vi "Ballard - 1553 - Message.vi"(8 "error in (no error)":errorcluster, 11 "Node Ptr":T2 format="%.0x") -> (0 "error out":errorcluster)   [LabVIEW 2020, in "Ballard 1553 System Explorer.lvlib"]
uses:
  Ballard 1553 System Explorer.lvlib
  <vilib>/NI VeriStand/Custom Device API/Custom Device API.lvlib
  Shared/Controls and Global/Global.vi
  Shared/Ballard 1553 Shared.lvlib
  SubVIs/Parse XML Ballard/Ballard_messageType.ctl
  <vilib>/NI VeriStand/Custom Device API/Get Item Property (Variant).vi
  SubVIs/Parse XML Ballard/Ballard_CWD1.ctl
  SubVIs/Parse XML Ballard/Ballard_CWD2.ctl
  <vilib>/NI VeriStand/Custom Device API/Get Item Property (U16).vi
  <vilib>/NI VeriStand/Custom Device API/Custom Device Item Ref.ctl
panel:
  out "TA2":i8 caption="Terminal Address (TA 2)"
  out "SA2":i8 caption="Terminal Sub-Address (SA 2)"
  out "MC":i8 caption="Mode Code (MC)"
  out "WC":i8 caption="Words Count (WC)"
  out "SA1":i8 caption="Terminal Sub-Address (SA 1)"
  out "TA1":i8 caption="Terminal Address (TA 1)"
  out "Message Type":T1
  in  "Header":cluster{"Section Name":string}={"Section Name"="Ballard - MIL-STD-1553 - Custom Device - Message"}
  in  "Description":string
  out "Name":string
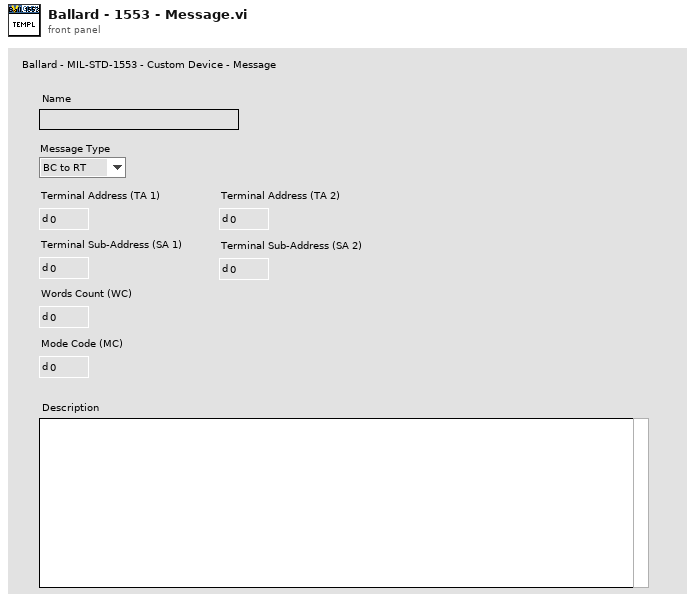
[diagram p1: front panel]
types:
  T1 = typedef "Ballard 1553 System Explorer.lvlib/Ballard_messageType.ctl" = enum16{"BC to RT", "RT to BC", "RT to RT", "MC (Rx)", "MC (Tx)"}
  T2 = typedef "Custom Device API.lvlib/Custom Device Item Ref.ctl" = u64
  T3 = typedef "Ballard 1553 System Explorer.lvlib/Ballard_CWD2.ctl" = cluster{"TA (RT)":i8, "SA":i8, "Words (WC)":i8}
  T4 = typedef "Ballard 1553 System Explorer.lvlib/Ballard_CWD1.ctl" = cluster{"TA (RT)":i8, "SA":i8, "Mode Code":i8, "Words Count":i8}
  T5 = typedef "Custom Device API.lvlib/Custom Device Item Info.ctl" = cluster{"Name":string, "Is Channel":bool, "GUID":string, "Is Waveform":bool}
  T6 = typedef "Custom Device API.lvlib/Custom Device Commands.ctl" = enum16{"Default", "Item renamed", "Shutdown", "Dynamic button pressed"}
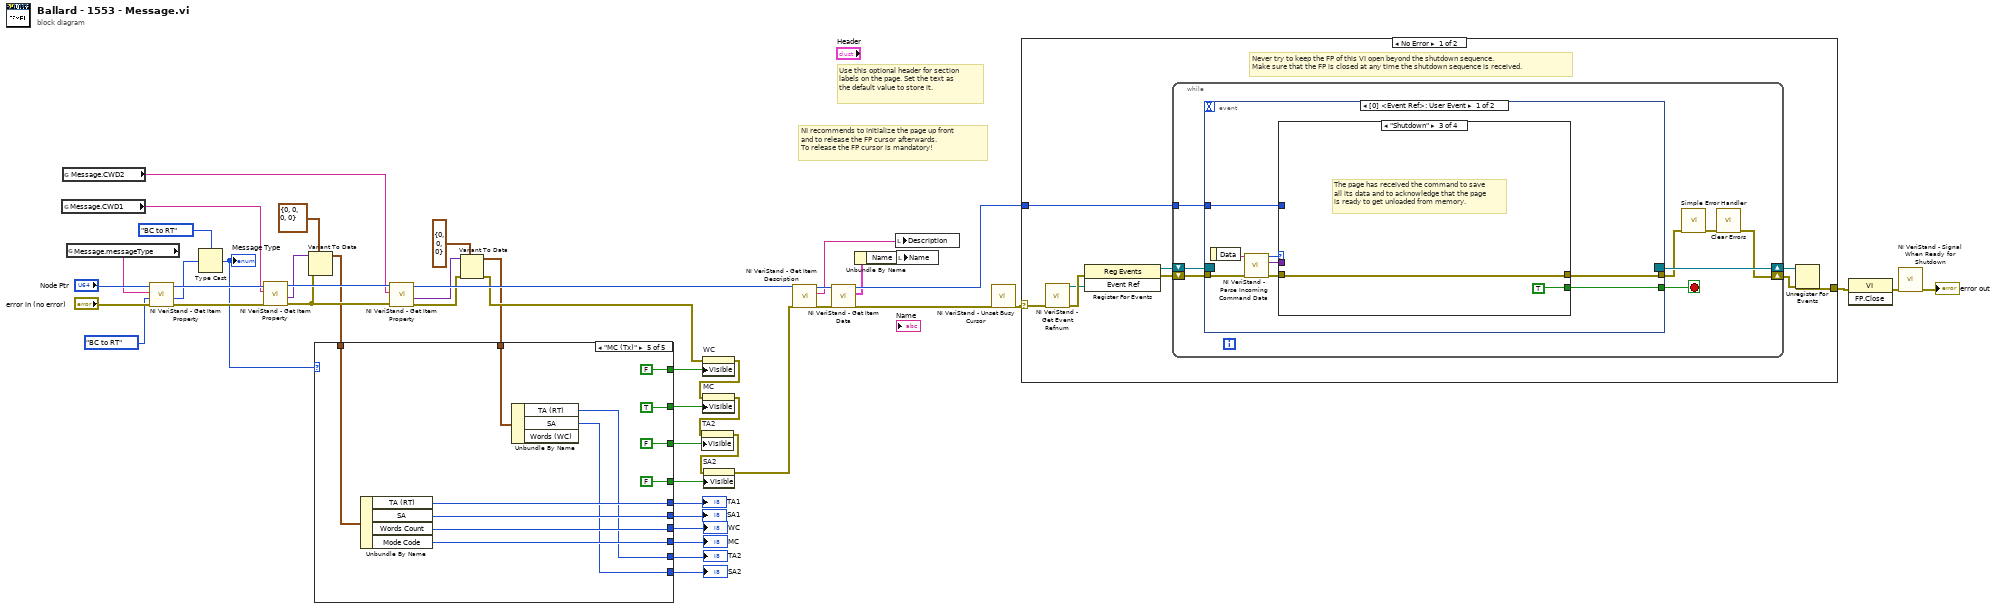
[diagram p0: block diagram]
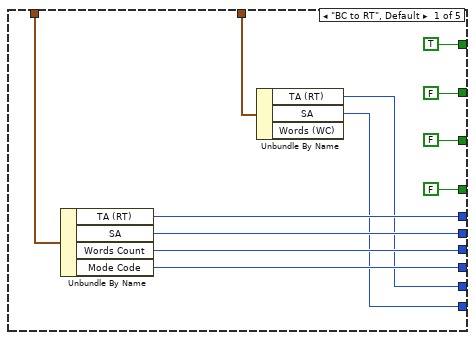
[diagram p2: hidden frame]
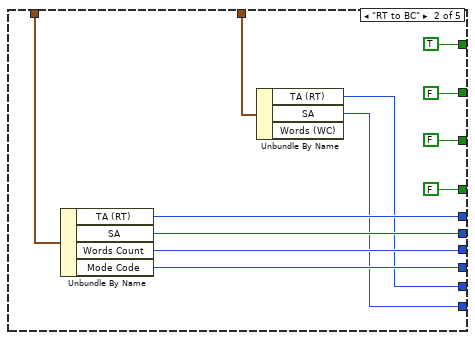
[diagram p3: hidden frame]
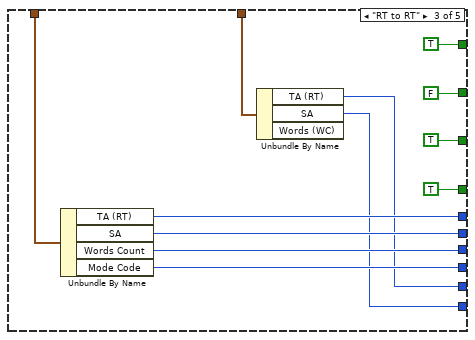
[diagram p4: hidden frame]
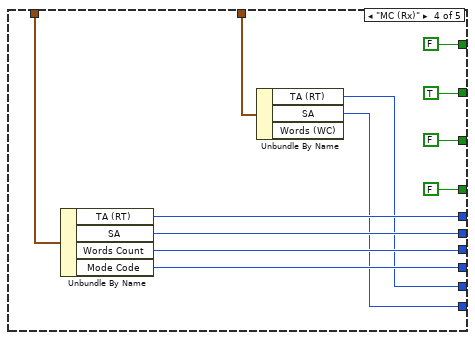
[diagram p5: hidden frame]
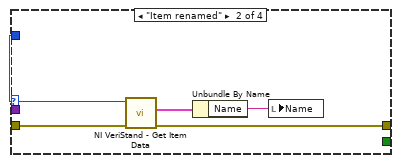
[diagram p7: hidden frame]
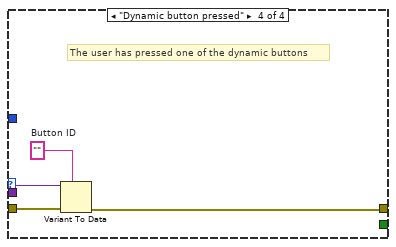
[diagram p8: hidden frame]
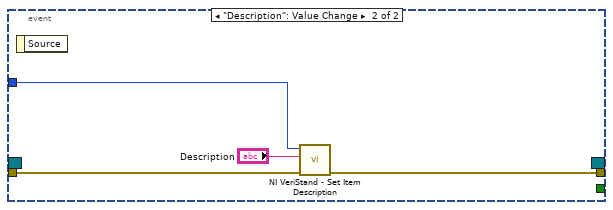
[diagram p9: hidden frame]
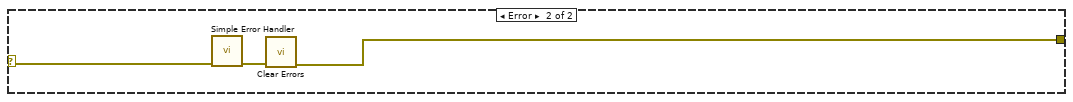
[diagram p10: hidden frame]
diagram:
  # "Use this optional header for section labels on the page. Set the text as the default value to store it."
  # "NI recommends to initialize the page up front\nand to release the FP cursor afterwards.\nTo release the FP cursor is mandatory!"
  n1 = global read "Global.vi" "Message.CWD1"() -> (w27:string)
  n2 = global read "Global.vi" "Message.CWD2"() -> (w21:string)
  n3 = global read "Global.vi" "Message.messageType"() -> (w31:string)
  n4 = call-poly <vilib>:"NI VeriStand - Get Item Property.vi"("error in (no error)"="error in (no error)", "Default Value"=Ballard_messageType."BC to RT" ("messageType"), "Property Name"=w31, "Item Ref in"="Node Ptr") -> ("error out"=w35:errorcluster, "Value"=w30:u16, "Item Ref out"=w32:T2)  [unwired: 4 in, 1 out]
  n5 = Type Cast(type=Ballard_messageType."BC to RT" ("messageType"), x=w30) -> (*(type *) &x=w18:T1)
  "Message Type" <- w18
  n6 = call-poly <vilib>:"NI VeriStand - Get Item Property.vi"("error in (no error)"=w35, "Property Name"=w27, "Item Ref in"=w32) -> ("error out"=w26:errorcluster, "Value"=w25:variant, "Item Ref out"=w36:T2)  [unwired: 5 in, 1 out]
  n7 = Variant To Data(error in=w26, type=T4 {"TA (RT)"=0, "SA"=0, "Mode Code"=0, "Words Count"=0} ("CWD1"), Variant=w25) -> (data=w12:T4)  [unwired: 1 out]
  n8 = call-poly <vilib>:"NI VeriStand - Get Item Property.vi"("error in (no error)"=w26, "Property Name"=w21, "Item Ref in"=w36) -> ("error out"=w20:errorcluster, "Value"=w19:variant, "Item Ref out"=w23:T2)  [unwired: 5 in, 1 out]
  n9 = Variant To Data(error in=w20, type=T3 {"TA (RT)"=0, "SA"=0, "Words (WC)"=0} ("CWD1"), Variant=w19) -> (data=w11:T3, error out=w17:errorcluster)
  n10 = case shown="\"MC (Tx)\"" w18 {
    tunnel: w12 -> [w55 w67 w79 w91 w103]
    tunnel: w11 -> [w50 w62 w74 w86 w98]
    tunnel: [FALSE FALSE TRUE FALSE FALSE] -> w10
    tunnel: [FALSE FALSE TRUE FALSE FALSE] -> w9
    tunnel: [FALSE FALSE FALSE TRUE TRUE] -> w8
    tunnel: [TRUE TRUE TRUE FALSE FALSE] -> w7
    tunnel: [w54 w66 w78 w90 w102] -> w6
    tunnel: [w53 w65 w77 w89 w101] -> w5
    tunnel: [w52 w64 w76 w88 w100] -> w4
    tunnel: [w51 w63 w75 w87 w99] -> w3
    tunnel: [w49 w61 w73 w85 w97] -> w2
    tunnel: [w48 w60 w72 w84 w96] -> w1
    frame "BC to RT", Default {
      n11 = Unbundle By Name(w55) -> ("TA (RT)"=w54:i8, "SA"=w53:i8, "Words Count"=w52:i8, "Mode Code"=w51:i8)
      n12 = Unbundle By Name(w50) -> ("TA (RT)"=w49:i8, "SA"=w48:i8)  [unwired: 1 out]
    }
    frame "RT to BC" {
      n13 = Unbundle By Name(w67) -> ("TA (RT)"=w66:i8, "SA"=w65:i8, "Words Count"=w64:i8, "Mode Code"=w63:i8)
      n14 = Unbundle By Name(w62) -> ("TA (RT)"=w61:i8, "SA"=w60:i8)  [unwired: 1 out]
    }
    frame "RT to RT" {
      n15 = Unbundle By Name(w79) -> ("TA (RT)"=w78:i8, "SA"=w77:i8, "Words Count"=w76:i8, "Mode Code"=w75:i8)
      n16 = Unbundle By Name(w74) -> ("TA (RT)"=w73:i8, "SA"=w72:i8)  [unwired: 1 out]
    }
    frame "MC (Rx)" {
      n17 = Unbundle By Name(w91) -> ("TA (RT)"=w90:i8, "SA"=w89:i8, "Words Count"=w88:i8, "Mode Code"=w87:i8)
      n18 = Unbundle By Name(w86) -> ("TA (RT)"=w85:i8, "SA"=w84:i8)  [unwired: 1 out]
    }
    frame "MC (Tx)" {
      n19 = Unbundle By Name(w103) -> ("TA (RT)"=w102:i8, "SA"=w101:i8, "Words Count"=w100:i8, "Mode Code"=w99:i8)
      n20 = Unbundle By Name(w98) -> ("TA (RT)"=w97:i8, "SA"=w96:i8)  [unwired: 1 out]
    }
  }
  "TA1" <- w6
  "SA1" <- w5
  "WC" <- w4
  "MC" <- w3
  "TA2" <- w2
  "SA2" <- w1
  n21 = property on="WC" class="DigNum (strict)"(error in=w17, "Visible"=w7) -> (error out=w16:errorcluster)  [unwired: 1 in, 1 out]
  n22 = property on="MC" class="DigNum (strict)"(error in=w16, "Visible"=w8) -> (error out=w15:errorcluster)  [unwired: 1 in, 1 out]
  n23 = property on="TA2" class="DigNum (strict)"(error in=w15, "Visible"=w10) -> (error out=w14:errorcluster)  [unwired: 1 in, 1 out]
  n24 = property on="SA2" class="DigNum (strict)"(error in=w14, "Visible"=w9) -> (error out=w13:errorcluster)  [unwired: 1 in, 1 out]
  n25 = call <vilib>:"NI VeriStand - Get Item Description.vi"("error in (no error)"=w13, "Item Ref in"=w23) -> ("error out"=w39:errorcluster, "Description"=w40:string, "Item Ref out"=w41:T2)  [unwired: 7 out]
  n26 = call <vilib>:"NI VeriStand - Get Item Data.vi"("error in (no error)"=w39, "Item Ref in"=w41) -> ("error out"=w44:errorcluster, "Item Info"=w38:T5, "Item Ref out"=w42:T2)  [unwired: 7 out]
  n27 = Unbundle By Name(w38) -> ("Name"=w37:string)
  n28 = local write "Description"(w40) -> ()
  n29 = local write "Name"(w37) -> ()
  n30 = call <vilib>:"NI VeriStand - Unset Busy Cursor.vi"("error in (no error)"=w44) -> ("error out"=w43:errorcluster)  [unwired: 10 out]
  n31 = case shown="No Error" w43 {
    selector: w43 -> [w108 w151]
    tunnel: [w113 w149] -> w47
    tunnel: w42 -> [w109 _]
    frame No Error {
      # "Never try to keep the FP of this VI open beyond the shutdown sequence.\nMake sure that the FP is closed at any time the shutdown sequence is received."
      n32 = call <vilib>:"NI VeriStand - Get Event Refnum.vi"("error in (no error)"=w108) -> ("error out"=w116:errorcluster, "Event Ref"=w112:refnum<user-event>)  [unwired: 9 out]
      n33 = register-events(error in=w116, w112) -> (reference out=w110:refnum<event-registration>, error out=w111:errorcluster)  [unwired: 1 in]
      n34 = while {
        tunnel: w109 -> [w120]
        shift-right: [w117] -> w114
        shift-left: w111 -> [w123]
        shift-right: [w124] -> w115
        shift-left: w110 -> [w122]
        stop <- w121 stop-if-true
        n35 = event shown="[0] <Event Ref>: User Event" {
          selector: w122 -> [_ _]
          dyn-events: [_ _] -> w124
          timeout: _ -> [_ _]
          tunnel: w123 -> [w132 w147]
          tunnel: [w128 _] -> w121
          tunnel: [w127 w146] -> w119
          tunnel: w120 -> [w126 w148]
          event User Event {
            n36 = event-data() -> ("Data"=w131:string)  [unwired: 1 out]
            n37 = call <vilib>:"NI VeriStand - Parse Incoming Command Data.vi"("error in (no error)"=w132, "Incoming data"=w131) -> ("error out"=w130:errorcluster, "Outgoing data"=w125:variant, "Action"=w129:T6)  [unwired: 7 out]
            n38 = case shown="\"Shutdown\"" w129 {
              tunnel: w130 -> [w133 w138 w139 w144]
              tunnel: [_ _ TRUE _] -> w128
              tunnel: [w133 w135 w139 w141] -> w127
              tunnel: w126 -> [_ w137 _ _]
              tunnel: w125 -> [_ _ _ w143]
              frame "Default", Default {
              }
              frame "Item renamed" {
                n39 = call <vilib>:"NI VeriStand - Get Item Data.vi"("error in (no error)"=w138, "Item Ref in"=w137) -> ("error out"=w135:errorcluster, "Item Info"=w136:T5)  [unwired: 8 out]
                n40 = Unbundle By Name(w136) -> ("Name"=w134:string)
                n41 = local write "Name"(w134) -> ()
              }
              frame "Shutdown" {
                # "The page has received the command to save all its data and to acknowledge that the page is ready to get unloaded from memory."
              }
              frame "Dynamic button pressed" {
                w142 = ""  # Button ID
                # "The user has pressed one of the dynamic buttons"
                n42 = Variant To Data(error in=w144, type=w142, Variant=w143) -> (error out=w141:errorcluster)  [unwired: 1 out]
              }
            }
          }
          event "Description": Value Change {
            n43 = event-data() -> ()  [unwired: 2 out]
            n44 = call <vilib>:"NI VeriStand - Set Item Description.vi"("error in (no error)"=w147, "Description"="Description", "Item Ref in"=w148) -> ("error out"=w146:errorcluster)  [unwired: 8 out]
          }
        }
        n45 = call <vilib>:"Simple Error Handler.vi"("error in (no error)"=w119) -> ("error out"=w118:errorcluster)  [unwired: 1 in, 7 out]
        n46 = call <vilib>:"Clear Errors.vi"("error in (no error)"=w118) -> ("error out"=w117:errorcluster)  [unwired: 1 in, 5 out]
      }
      n47 = Unregister For Events(event registration refnum=w115, error in=w114) -> (error out=w113:errorcluster)
    }
    frame Error {
      n48 = call <vilib>:"Simple Error Handler.vi"("error in (no error)"=w151) -> ("error out"=w150:errorcluster)  [unwired: 1 in, 7 out]
      n49 = call <vilib>:"Clear Errors.vi"("error in (no error)"=w150) -> ("error out"=w149:errorcluster)  [unwired: 1 in, 5 out]
    }
  }
  n50 = invoke class="VI" method="FP.Close"(error in=w47) -> (error out=w46:errorcluster)  [unwired: 2 in, 2 out]
  n51 = call <vilib>:"NI VeriStand - Signal When Ready for Shutdown.vi"("error in (no error)"=w46) -> ("error out"=→"error out":errorcluster)  [unwired: 10 out]
